vi "PDCGetAllLists.vi"(0 "DeviceNo":u32, 5 "ChildNo":u32, 11 "error in (no error)":errorcluster) -> (4 "ResolutionList":string[](array[string]), 6 "RecordRateList":string[](array[string]), 8 "ShutterSpeedList":string[](array[string]), 10 "TriggerModeList":string[](array[string]), 15 "error out":errorcluster)   [LabVIEW 2015]
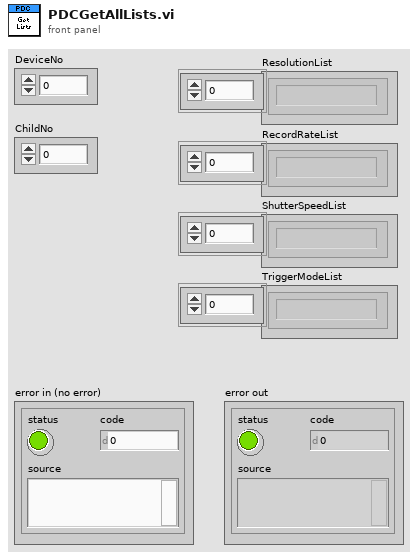
[diagram p1: front panel]
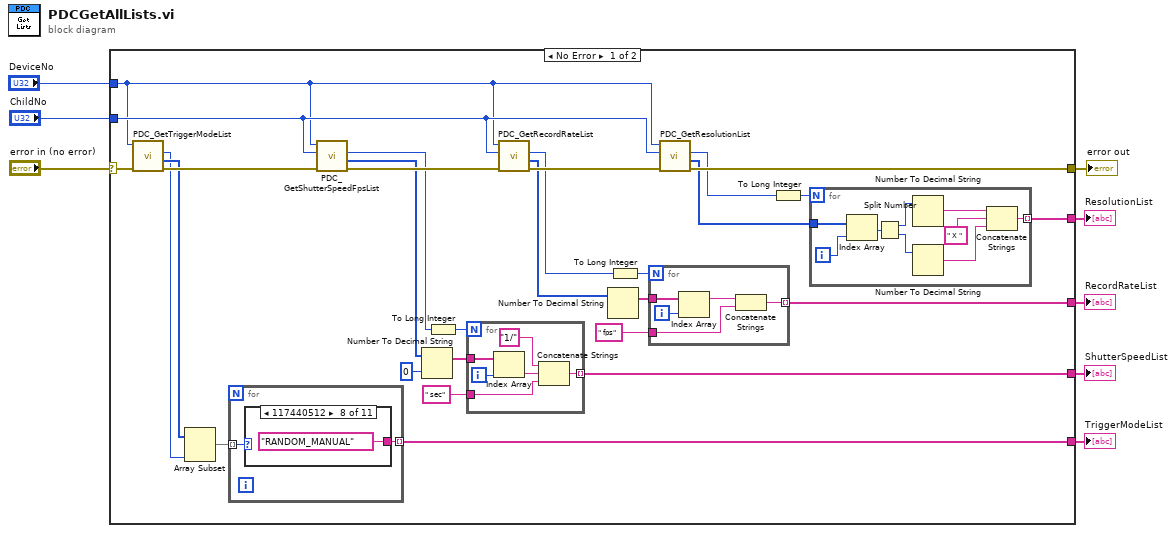
[diagram p0: block diagram]
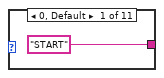
[diagram p2: hidden frame]
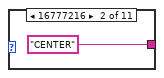
[diagram p3: hidden frame]
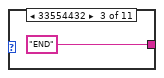
[diagram p4: hidden frame]
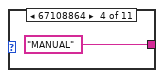
[diagram p5: hidden frame]
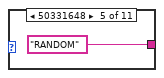
[diagram p6: hidden frame]
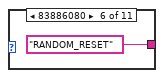
[diagram p7: hidden frame]
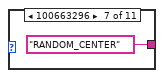
[diagram p8: hidden frame]
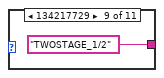
[diagram p9: hidden frame]
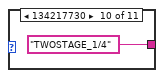
[diagram p10: hidden frame]
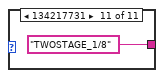
[diagram p11: hidden frame]
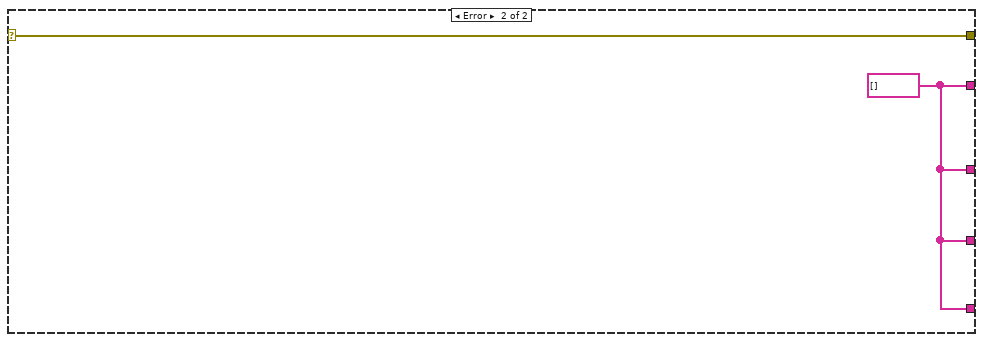
[diagram p12: hidden frame]
diagram:
  n1 = case shown="No Error" "error in (no error)" {
    selector: "error in (no error)" -> [w15 w71]
    tunnel: [w36 w71] -> w8
    tunnel: "DeviceNo" -> [w13 _]
    tunnel: "ChildNo" -> [w25 _]
    tunnel: [w18 w70] -> w4
    tunnel: [w17 w70] -> w3
    tunnel: [w16 w70] -> w2
    tunnel: [w12 w70] -> w1
    frame No Error {
      n2 = call "PDC_GetTriggerModeList.vi"("error in (no error)"=w15, "DeviceNo"=w13) -> ("error out"=w14:errorcluster, "List"=w11:u32[], "Size"=w9:u32)  [unwired: 5 in, 2 out]
      n3 = Array Subset(array=w11, length=w9) -> (w10:u32[])  [unwired: 1 in]
      n4 = for {
        tunnel: [w38] -> w12 mode=indexing
        tunnel: w10 -> [w37] mode=indexing
        n5 = case shown="117440512" w37 {
          tunnel: ["START" "CENTER" "END" "MANUAL" "RANDOM" "RANDOM_RESET" "RANDOM_CENTER" "RANDOM_MANUAL" "TWOSTAGE_1/2" "TWOSTAGE_1/4" "TWOSTAGE_1/8"] -> w38
          frame 0, Default {
          }
          frame 16777216 {
          }
          frame 33554432 {
          }
          frame 67108864 {
          }
          frame 50331648 {
          }
          frame 83886080 {
          }
          frame 100663296 {
          }
          frame 117440512 {
          }
          frame 134217729 {
          }
          frame 134217730 {
          }
          frame 134217731 {
          }
        }
      }
      n6 = call "PDC_GetShutterSpeedFpsList.vi"("error in (no error)"=w14, "ChildNo"=w25, "DeviceNo"=w13) -> ("error out"=w35:errorcluster, "List"=w21:u32[], "Size"=w19:u32)  [unwired: 4 in, 2 out]
      n7 = Number To Decimal String(number=w21, width (-)=u32 0 ("i-j")) -> (decimal integer string=w22:string[])
      n8 = To Long Integer(number=w19) -> (32bit integer=w20:i32)
      n9 = for {
        N: w20 -> [_]
        tunnel: w22 -> [w54]
        tunnel: [w55] -> w16 mode=indexing
        tunnel: " sec" -> [w51]
        i -> [w53]
        n10 = Index Array(array=w54, index=w53) -> (element=w52:string)
        n11 = Concatenate Strings("1/", w52, w51) -> (w55:string)
      }
      n12 = call "PDC_GetResolutionList.vi"("error in (no error)"=w35, "ChildNo"=w25, "DeviceNo"=w13) -> ("error out"=w34:errorcluster, "List"=w26:u32[], "Size"=w28:u32)  [unwired: 4 in, 2 out]
      n13 = call "PDC_GetRecordRateList.vi"("error in (no error)"=w34, "ChildNo"=w25, "DeviceNo"=w13) -> ("error out"=w36:errorcluster, "List"=w33:u32[], "Size"=w31:u32)  [unwired: 4 in, 2 out]
      n14 = Number To Decimal String(number=w33) -> (decimal integer string=w30:string[])  [unwired: 1 out]
      n15 = To Long Integer(number=w31) -> (32bit integer=w32:i32)
      n16 = for {
        N: w32 -> [_]
        tunnel: w30 -> [w58]
        tunnel: [w60] -> w17 mode=indexing
        tunnel: " fps" -> [w59]
        i -> [w57]
        n17 = Index Array(array=w58, index=w57) -> (element=w56:string)
        n18 = Concatenate Strings(w56, w59) -> (w60:string)
      }
      n19 = To Long Integer(number=w28) -> (32bit integer=w27:i32)
      n20 = for {
        N: w27 -> [_]
        tunnel: [w67] -> w18 mode=indexing
        tunnel: w26 -> [w66]
        i -> [w65]
        n21 = Index Array(array=w66, index=w65) -> (element=w64:u32)
        n22 = Split Number(x=w64) -> (hi(x)=w63:u16, lo(x)=w62:u16)
        n23 = Number To Decimal String(number=w63) -> (decimal integer string=w69:string)  [unwired: 1 out]
        n24 = Number To Decimal String(number=w62) -> (decimal integer string=w68:string)  [unwired: 1 out]
        n25 = Concatenate Strings(w69, " X ", w68) -> (w67:string)
      }
    }
    frame Error {
      w70 = string[] []
    }
  }
  "error out" <- w8
  "ResolutionList" <- w4
  "RecordRateList" <- w3
  "ShutterSpeedList" <- w2
  "TriggerModeList" <- w1
